vi "VHQueryHostBitness.vi"(8 "error in (no error)":errorcluster) -> (0 "error out":errorcluster, 2 "Is 64 bit":bool)   [LabVIEW 2013, in "VIHost.lvlib"]
uses:
  VIHost.lvlib
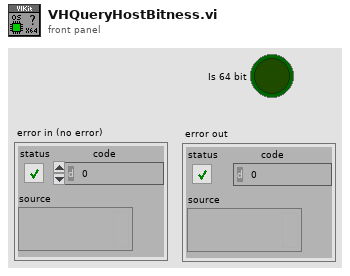
[diagram p1: front panel]
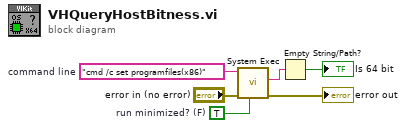
[diagram p0: block diagram]
diagram:
  w5 = TRUE  # run minimized? (F)
  w6 = "cmd /c set programfiles(x86)"  # command line
  n1 = call <vilib>:"System Exec.vi"("run minimized? (F)"=w5, "error in (no error)"="error in (no error)", "command line"=w6) -> ("error out"=→"error out":errorcluster, "standard error"=w3:string)  [unwired: 5 in, 2 out]
  n2 = Empty String/Path?(string/path=w3) -> (empty?=→"Is 64 bit":bool)
